vi "Get Aircraft RX Queue String.vi"(8 "Error In":errorcluster, 11 "Aircraft ID":u8) -> (0 "Error Out":errorcluster, 3 "Aircraft Q Name":string)   [LabVIEW 2014]
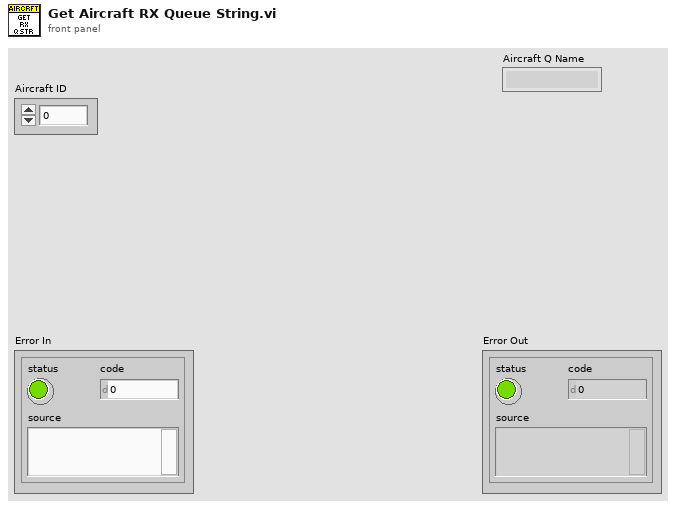
[diagram p1: front panel]
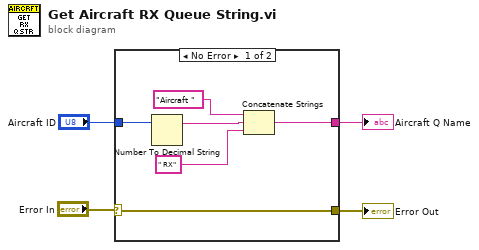
[diagram p0: block diagram]
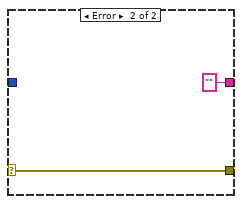
[diagram p2: hidden frame]
diagram:
  n1 = case shown="No Error" "Error In" {
    selector: "Error In" -> [w5 w11]
    tunnel: "Aircraft ID" -> [w9 _]
    tunnel: [w6 ""] -> w3
    tunnel: [w5 w11] -> w1
    frame No Error {
      n2 = Number To Decimal String(number=w9) -> (decimal integer string=w8:string)  [unwired: 1 in]
      n3 = Concatenate Strings("Aircraft ", w8, " RX" ("string")) -> (w6:string)
    }
    frame Error {
    }
  }
  "Aircraft Q Name" <- w3
  "Error Out" <- w1
